vi "Points Difference.vi"(1 "포인트 개수(소비자 루프)":i32, 2 "놓친 포인트 컨트롤 참조 번호":refnum<vi>, 3 "포인트 개수(생산자 루프)":i32) -> (0 "놓친 포인트":i32)   [LabVIEW 2011]
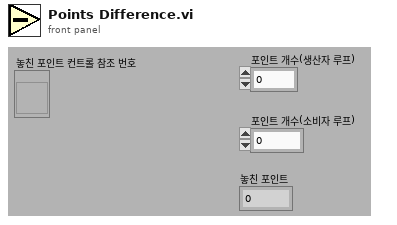
[diagram p1: front panel]
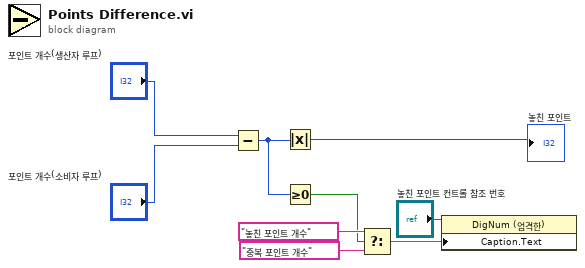
[diagram p0: block diagram]
diagram:
  n1 = Subtract(x="포인트 개수(생산자 루프)", y="포인트 개수(소비자 루프)") -> (x-y=w8:i32)
  n2 = Absolute Value(x=w8) -> (abs(x)=→"놓친 포인트":i32)
  n3 = Greater Or Equal To 0?(x=w8) -> (x >= 0?=w4:bool)
  n4 = Select(t="놓친 포인트 개수", s=w4, f="중복 포인트 개수") -> (s? t:f=w7:string)
  n5 = property on="Property Node" class="DigNum (엄격한)"(reference="놓친 포인트 컨트롤 참조 번호", "Caption.Text"=w7) -> ()  [unwired: 1 in, 2 out]
